vi "Initialize KUKA youBot Gripper.vi"(8 "error in (no error)":errorcluster, 11 "KUKA youBot gripper in":refnum<class "NI_Robotics_KUKA youBot Gripper.lvclass">) -> (0 "error out":errorcluster, 3 "KUKA youBot gripper out":refnum<class "NI_Robotics_KUKA youBot Gripper.lvclass">)   [LabVIEW 2017, in "NI_Robotics_KUKA youBot Host.lvlib" / "NI_Robotics_KUKA youBot Gripper.lvclass"]
uses:
  <vilib>/robotics/KUKA youBot/Basic Device/Gripper/NI_Robotics_KUKA youBot Gripper.lvclass
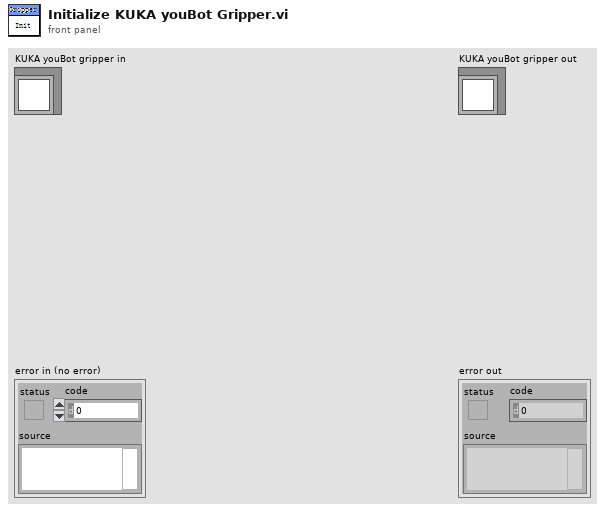
[diagram p1: front panel]
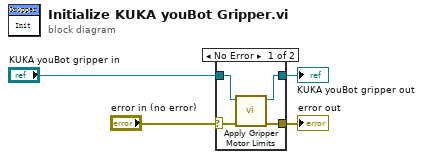
[diagram p0: block diagram]
diagram:
  n1 = case shown="No Error" "error in (no error)" {
    selector: "error in (no error)" -> [w6 w10]
    tunnel: [w5 w10] -> w3
    tunnel: [w7 w9] -> w1
    tunnel: "KUKA youBot gripper in" -> [w8 w9]
    frame No Error {
      n2 = call <vilib>:"Apply Gripper Motor Limits.vi"("error in (no error)"=w6, "KUKA youBot gripper in"=w8) -> ("error out"=w5:errorcluster, "KUKA youBot gripper out"=w7:refnum<class "NI_Robotics_KUKA youBot Gripper.lvclass">)  [unwired: 8 in]
    }
    frame Error {
    }
  }
  "error out" <- w3
  "KUKA youBot gripper out" <- w1
